vi "XLP80_Datalog_GetDataString.vi"(8 "error in":errorcluster, 11 "Comment":string) -> (0 "error OUT":errorcluster caption="error out", 2 "String":string)   [LabVIEW 2021]
doc: "Speichert die aktuelle Zeit und die aktuellen Daten im File ab."
uses:
  XLP80_General_Libs/WL_Libs_V14.25/WL_Datalog_V14.00.llb/WL_Datalog_Global.vi
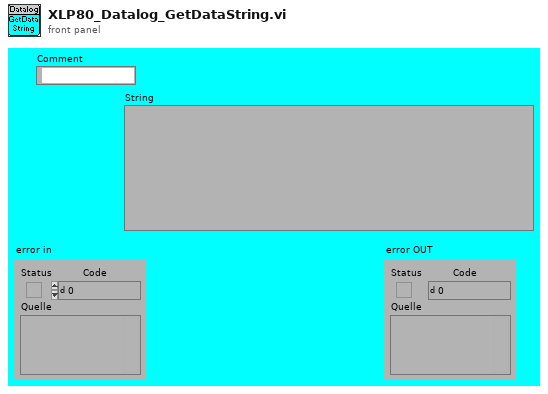
[diagram p1: front panel]
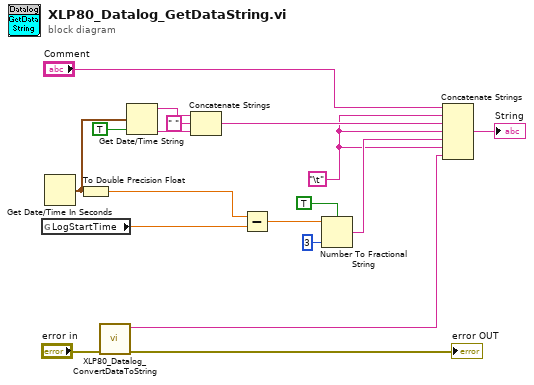
[diagram p0: block diagram]
diagram:
  w1 = "\t" ("Substring")
  n1 = global read "WL_Datalog_Global.vi" "LogStartTime"() -> (w5:dbl)
  n2 = Get Date/Time In Seconds() -> (seconds since 1Jan1904=w3:timestamp)
  n3 = To Double Precision Float(number=w3) -> (double precision float=w4:dbl)
  n4 = call "XLP80_Datalog_ConvertDataToString.vi"("error in"="error in") -> ("error OUT"=→"error OUT":errorcluster, "DataString"=w2:string)  [unwired: 9 in]
  n5 = Get Date/Time String(seconds (now)=w3, want seconds? (F)=TRUE) -> (date string=w15:string, time string=w12:string)  [unwired: 1 in]
  n6 = Concatenate Strings(w15, " " ("Substring"), w12) -> (w14:string)
  n7 = Subtract(x=w4, y=w5) -> (x-y=w8:dbl)
  n8 = Number To Fractional String(use system decimal point (T)=TRUE, number=w8, precision (6)=i16 3) -> (F-format string=w10:string)  [unwired: 1 in]
  n9 = Concatenate Strings("Comment", w1, w14, w1, w10, w1, w2) -> (→"String":string)
